vi "Selected items.vi"(10 "Item Syms":i32[](array[numeric]), 11 "Item name":string[](array[string])) -> (1 "Selected tem index":i32[](array[numeric]), 2 "Item Seleced?":bool, 3 "Selected tem":string[](array[string]))   [LabVIEW 2011]
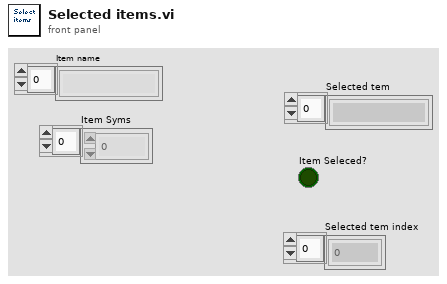
[diagram p1: front panel]
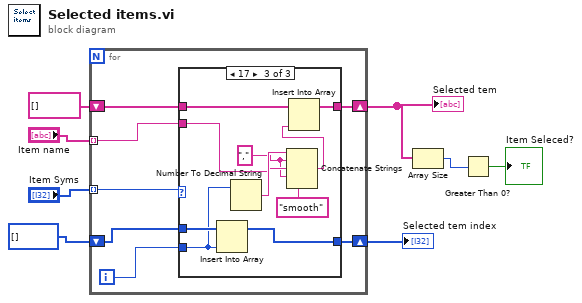
[diagram p0: block diagram]
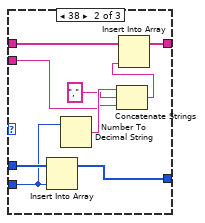
[diagram p3: hidden frame]
diagram:
  n1 = for {
    tunnel: "Item name" -> [w14] mode=indexing
    tunnel: "Item Syms" -> [w9] mode=indexing
    shift-right: [w13] -> w5
    shift-left: string[] [] ("Item name") -> [w15]
    shift-right: [w10] -> w1
    shift-left: i32[] [] ("Item Syms") -> [w12]
    i -> [w11]
    n2 = case shown="17" w9 {
      tunnel: w15 -> [w17 w26 w36]
      tunnel: w14 -> [_ w20 w31]
      tunnel: [w17 w21 w32] -> w13
      tunnel: w12 -> [w16 w25 w35]
      tunnel: w11 -> [_ w18 w29]
      tunnel: [w16 w24 w34] -> w10
      frame 37, Default {
      }
      frame 38 {
        n3 = Insert Into Array(array=w25, new element=w18) -> (w24:i32[])  [unwired: 1 in]
        n4 = Number To Decimal String(number=w18) -> (decimal integer string=w23:string)  [unwired: 1 in]
        n5 = Concatenate Strings(w23, "," ("字符串"), w20) -> (w19:string)
        n6 = Insert Into Array(array=w26, new element=w19) -> (w21:string[])  [unwired: 1 in]
      }
      frame 17 {
        w28 = "," ("字符串")
        n7 = Insert Into Array(array=w35, new element=w29) -> (w34:i32[])  [unwired: 1 in]
        n8 = Number To Decimal String(number=w29) -> (decimal integer string=w33:string)  [unwired: 1 in]
        n9 = Concatenate Strings(w33, w28, w31, w28, "smooth" ("字符串")) -> (w30:string)
        n10 = Insert Into Array(array=w36, new element=w30) -> (w32:string[])  [unwired: 1 in]
      }
    }
  }
  "Selected tem" <- w5
  "Selected tem index" <- w1
  n11 = Array Size(array=w5) -> (size(s)=w3:i32)
  n12 = Greater Than 0?(x=w3) -> (x > 0?=→"Item Seleced?":bool)
